vi "Read configuration.vi"(8 "error in (no error)":errorcluster, 11 "Abstract Digitizer in":refnum<class "Digitizer Instrument.lvclass">) -> (0 "error out":errorcluster, 2 "configuration":refnum<class "CEF_serializable configuration.lvclass">, 3 "Abstract Digitizer out":refnum<class "Digitizer Instrument.lvclass">)   [LabVIEW 2025, in "Digitizer.lvlib" / "Digitizer Instrument.lvclass"]
uses:
  Digitizer Instrument.lvclass
  Users/Public/Documents/Sandia National Labs/TSS Plugin/CEF.lvlibp/serializable configuration/CEF_serializable configuration.lvclass
  Digitizer Instrument.lvclass/Digitizer Instrument.ctl
  Digitizer configuration/Digitizer configuration.lvclass
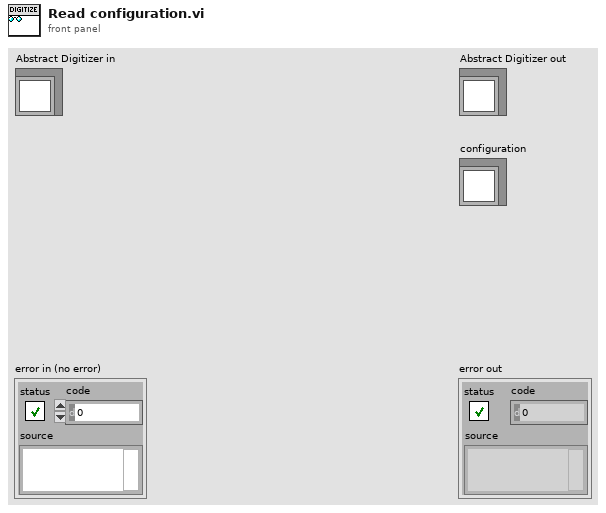
[diagram p1: front panel]
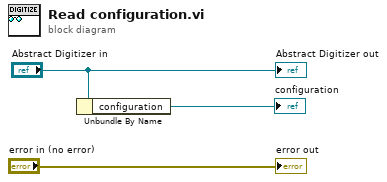
[diagram p0: block diagram]
diagram:
  n1 = Unbundle By Name("Abstract Digitizer in") -> ("configuration"=→"configuration":refnum<class "Digitizer configuration.lvclass">)
  "error out" <- "error in (no error)"
  "Abstract Digitizer out" <- "Abstract Digitizer in"
